vi "Change Audio Speed.vi"(11 "Audio Block":dbl[][](array[numeric])) -> (3 "Interpolated Audio":dbl[][](array[numeric]))   [LabVIEW 2019, in "Audio Processing.lvlib"]
doc: "Stretches or squashes the input audio block (via interpolation) to the fixed audio processing block size. This in effect changes the speed of the audio."
uses:
  Audio Processing.lvlib
  Globals/Constants.vi
  <vilib>/gmath/NI_Gmath.lvlib
  Globals/Globals.lvlib
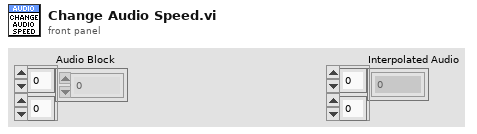
[diagram p1: front panel]
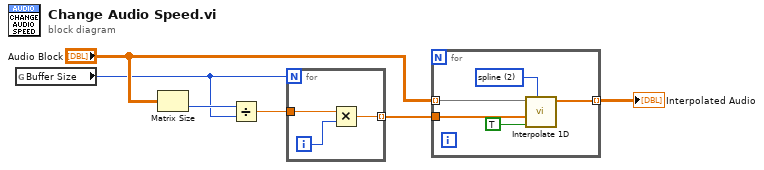
[diagram p0: block diagram]
diagram:
  n1 = global read "Constants.vi" "Buffer Size"() -> (w1:i32)
  n2 = Matrix Size(0:"Audio Block") -> (2:w3:i32)  [unwired: 1 out]
  n3 = Divide(x=w3, y=w1) -> (x/y=w2:dbl)
  n4 = for {
    N: w1 -> [_]
    tunnel: w2 -> [w8]
    tunnel: [w7] -> w6 mode=indexing
    i -> [w9]
    n5 = Multiply(x=w8, y=w9) -> (x*y=w7:dbl)
  }
  n6 = for {
    tunnel: "Audio Block" -> [w14] mode=indexing
    tunnel: w6 -> [w12]
    tunnel: [w10] -> w5 mode=indexing
    w11 = 2 items=["nearest", "linear", "spline", "cubic Hermite", "Lagrange"] ("method")
    n7 = call <vilib>:"Interpolate 1D.vi"("method"=w11, "X is monotonic"=TRUE, "xi"=w12, "Y"=w14) -> ("yi"=w10:dbl[])  [unwired: 5 in, 2 out]
  }
  "Interpolated Audio" <- w5
